vi "1.4-How.vi"   [LabVIEW 2010]
uses:
  2-Low Neurons/2.4-How Sensor Typedef.ctl
  <vilib>/eio/EIONode/EIONode.xnode
  <vilib>/rvi/eio/nirviEIOImplementation/nirviEIOImplementation.xnode
  <vilib>/rvi/eio/common/nirviEmuClasses.ctl
  1.0-Hindbrain Global.vi
  <vilib>/rvi/eio/common/nirviEmuTemplateMethod_noerrors.vi
types:
  T1 = typedef "2.4-How Sensor Typedef.ctl" = cluster{"Motor Speed Integer":i16, "Drive Position Integer":i32, "Lidar Position Integer":i32, "Steering Position Integer":i32, "Battery Voltage Fxp":fxp<+/-,16,5>, "Drive Control Voltage":fxp<+/-,20,5>, "Steering Control Voltage":fxp<+/-,20,5>, "Drive Encoder Cable Check":bool, "Lidar Drive Encoder Cable Check":bool, "Steer Encoder Cable Check":bool, "Lidar Pos Encoder Cable Check":bool, "Mod Buttons & Blinky Cable Check":bool, "Lidar Data Cable Check":bool, "Drive Motor Cable Check":bool, "Vector Nav Cable Check":bool, "Lidar Drive Cable Check":bool, "Steer Drive Cable Check":bool}
  T2 = typedef "nirviEmuClasses.ctl" = enum16{"IO Read", "IO Write", "Method", "Property Read", "Property Write"}
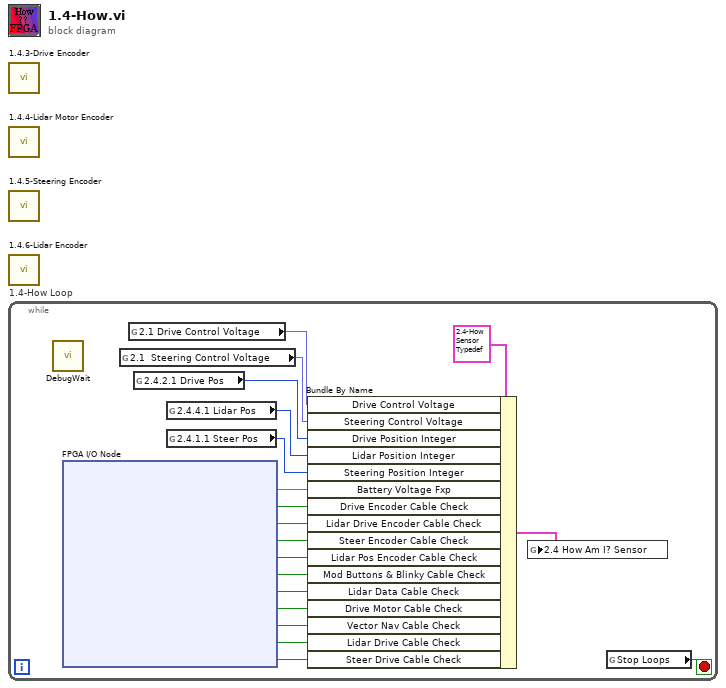
[diagram p0: block diagram]
diagram:
  n1 = call "1.4.3-Drive Encoder.vi"() -> ()  [unwired: 1 in]
  n2 = call "1.4.4-Lidar Motor Encoder.vi"() -> ()  [unwired: 1 in]
  n3 = call "1.4.5-Steering Encoder.vi"() -> ()  [unwired: 1 in]
  n4 = call "1.4.6-Lidar Encoder.vi"() -> ()  [unwired: 1 in]
  n5 = while "1.4-How Loop" {
    stop <- w19 stop-if-true
    n6 = call "DebugWait.vi"() -> ()  [unwired: 12 in]
    n7 = xnode "FPGA I/O Node"() -> ("Battery Voltage"=w14:fxp<+/-,16,5>, "Drive Encoder Cable Check"=w4:bool, "Lidar Drive Encoder Cable Check"=w5:bool, "Steer Encoder Cable Check"=w6:bool, "Lidar Pos Encoder Cable Check"=w7:bool, "Mod Btns + Blinky Cable Check"=w8:bool, "Lidar Data Cable Check"=w9:bool, "Drive Motor Cable Check"=w10:bool, "Vector Nav Cable Check"=w11:bool, "Lidar Drive Cable Check"=w12:bool, "Steer Drive Cable Check"=w13:bool)  [unwired: 11 in, 11 out]
    n8 = global read "1.0-Hindbrain Global.vi" "2.1  Steering Control Voltage"() -> (w3:fxp<+/-,20,5>)
    n9 = global read "1.0-Hindbrain Global.vi" "2.1 Drive Control Voltage"() -> (w2:fxp<+/-,20,5>)
    n10 = global read "1.0-Hindbrain Global.vi" "2.4.2.1 Drive Pos"() -> (w1:i32)
    n11 = global read "1.0-Hindbrain Global.vi" "2.4.4.1 Lidar Pos"() -> (w15:i32)
    n12 = global read "1.0-Hindbrain Global.vi" "2.4.1.1 Steer Pos"() -> (w16:i32)
    n13 = Bundle By Name(cluster=T1 {"Motor Speed Integer"=0, "Drive Position Integer"=0, "Lidar Position Integer"=0, "Steering Position Integer"=0, "Battery Voltage Fxp"=0.0, "Drive Control Voltage"=0.0, "Steering Control Voltage"=0.0, "Drive Encoder Cable Check"=FALSE, "Lidar Drive Encoder Cable Check"=FALSE, "Steer Encoder Cable Check"=FALSE, "Lidar Pos Encoder Cable Check"=FALSE, "Mod Buttons & Blinky Cable Check"=FALSE, "Lidar Data Cable Check"=FALSE, "Drive Motor Cable Check"=FALSE, "Vector Nav Cable Check"=FALSE, "Lidar Drive Cable Check"=FALSE, "Steer Drive Cable Check"=FALSE} ("2.4 How Am I? Sensor"), "Drive Control Voltage"=w2, "Steering Control Voltage"=w3, "Drive Position Integer"=w1, "Lidar Position Integer"=w15, "Steering Position Integer"=w16, "Battery Voltage Fxp"=w14, "Drive Encoder Cable Check"=w4, "Lidar Drive Encoder Cable Check"=w5, "Steer Encoder Cable Check"=w6, "Lidar Pos Encoder Cable Check"=w7, "Mod Buttons & Blinky Cable Check"=w8, "Lidar Data Cable Check"=w9, "Drive Motor Cable Check"=w10, "Vector Nav Cable Check"=w11, "Lidar Drive Cable Check"=w12, "Steer Drive Cable Check"=w13) -> (w17:T1)
    n14 = global write "1.0-Hindbrain Global.vi" "2.4 How Am I? Sensor"(w17) -> ()
    n15 = global read "1.0-Hindbrain Global.vi" "Stop Loops"() -> (w19:bool)
  }
